vi "main.vi"(8 "error in (no error)":errorcluster) -> (0 "error out":errorcluster)   [LabVIEW 2018]
doc: "Main VI."
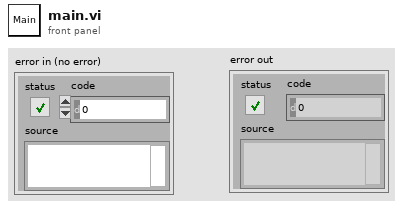
[diagram p1: front panel]
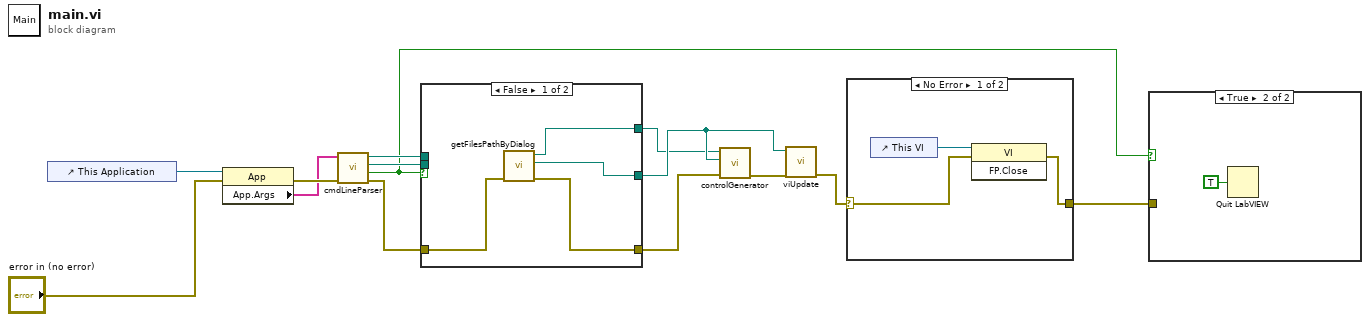
[diagram p0: block diagram]
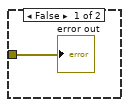
[diagram p2: hidden frame]
diagram:
  n1 = control-ref of="This Application"() -> (w4:refnum<vi>)
  n2 = property class="App"(reference=w4, error in="error in (no error)") -> (error out=w2:errorcluster, "App.Args"=w1:string[])  [unwired: 1 out]
  n3 = call "cmdLineParser.vi"("error in (no error)"=w2, "cmdLineArgs"=w1) -> ("error out"=w12:errorcluster, "filesExist"=w8:bool, "pathLvlibDir"=w10:path, "pathIdl"=w11:path)  [unwired: 6 in]
  n4 = case shown="False" w8 {
    tunnel: w12 -> [w18 w21]
    tunnel: [w17 w21] -> w6
    tunnel: [w16 w20] -> w5
    tunnel: [w15 w19] -> w9
    tunnel: w11 -> [_ w20]
    tunnel: w10 -> [_ w19]
    frame False {
      n5 = call "getFilesPathByDialog.vi"("error in (no error)"=w18) -> ("error out"=w17:errorcluster, "pathLvlibDir"=w15:path, "pathIdl"=w16:path)  [unwired: 8 in]
    }
    frame True {
    }
  }
  n6 = call "controlGenerator.vi"("error in (no error)"=w6, "ControlOutputPath"=w9, "ComponentIDLFile"=w5) -> ("error out"=w13:errorcluster)  [unwired: 8 in]
  n7 = call "viUpdate.vi"("error in (no error)"=w13, "OutputPath"=w9) -> ("error out"=w14:errorcluster)  [unwired: 9 in]
  n8 = case shown="No Error" w14 {
    selector: w14 -> [w22 w25]
    tunnel: [w23 w25] -> w7
    frame No Error {
      n9 = control-ref of="This VI"() -> (w24:refnum<vi>)
      n10 = invoke class="VI" method="FP.Close"(reference=w24, error in=w22) -> (error out=w23:errorcluster)  [unwired: 1 in, 2 out]
    }
    frame Error {
    }
  }
  n11 = case shown="True" w8 {
    tunnel: w7 -> [w26 _]
    frame False {
      "error out" <- w26
    }
    frame True {
      n12 = Quit LabVIEW(quit? (T)=TRUE) -> ()
    }
  }
